vi "Cmd Get Parameter Value.vi"(4 "error in (no error)":errorcluster, 6 "parameter index":variant, 7 "command reference":T1) -> (0 "error out":errorcluster, 1 "value":variant, 3 "command reference out":T1)   [LabVIEW 2012, in "NI_Database_API_64.lvlib"]
doc: "Returns the value of a specified parameter given the command reference. The <B>parameter index</B> can either be the zero-indexed position of the parameter in the command or the name of the parameter."
uses:
  NI_Database_API_64.lvlib
  Cmd ObjectReference.ctl
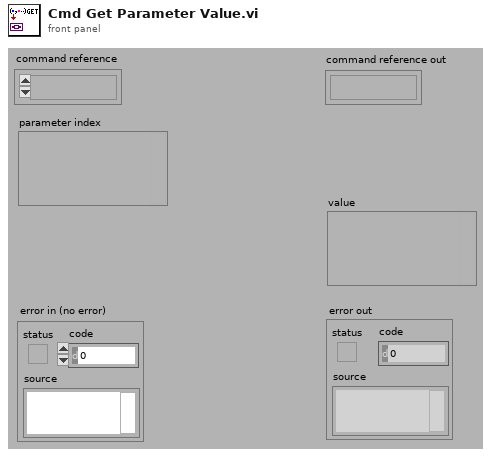
[diagram p1: front panel]
types:
  T1 = typedef "NI_Database_API_64.lvlib/Cmd ObjectReference.ctl" = refnum<k1>
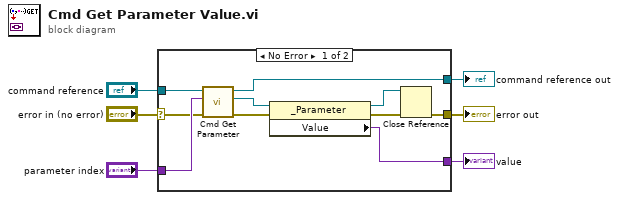
[diagram p0: block diagram]
diagram:
  n1 = case shown="No Error" "error in (no error)" {
    selector: "error in (no error)" -> [w7 w18]
    tunnel: [w15 _] -> w6
    tunnel: "command reference" -> [w13 w17]
    tunnel: "parameter index" -> [w12 _]
    tunnel: [w9 w18] -> w3
    tunnel: [w8 w17] -> w2
    frame No Error {
      n2 = call "Cmd Get Parameter.vi"("error in (no error)"=w7, "parameter index"=w12, "command reference"=w13) -> ("error out"=w16:errorcluster, "ADODB.Parameter"=w14:refnum<k7>, "command reference out"=w8:T1)  [unwired: 2 in]
      n3 = property class="_Parameter"(reference=w14, error in=w16) -> (reference out=w10:refnum<k7>, error out=w11:errorcluster, "Value"=w15:variant)
      n4 = Close Reference(reference=w10, error in (no error)=w11) -> (error out=w9:errorcluster)
    }
    frame Error {
    }
  }
  "value" <- w6
  "error out" <- w3
  "command reference out" <- w2
